vi "onStart.vi"(8 "error in (no error)":errorcluster, 11 "Camera":refnum<class "Camera.lvclass">) -> (0 "error out":errorcluster, 3 "Camera out":refnum<class "Camera.lvclass">)   [LabVIEW 2013, in "Camera.lvclass"]
doc: "JKI State Machine Objects (SMO) 1.0.4.18\nJKI - JKI\nCopyright (c) 2016, JKI"
uses:
  Camera.lvclass
  <vilib>/JKI/JKI SMO/SMO/SMO.lvclass
panel:
  # "For instructions on how to use the JKI State Machine Objects, examples and video tutorials, visit:\nhttp://jki.net/state-machine-objects/\n\nJKI State Machine Objects™\nhttp://jki.net/state-machine-objects/\nCopyright (C) 2005-2015, JKI <info@jki.net>\nALL RIGHTS RESERVED"
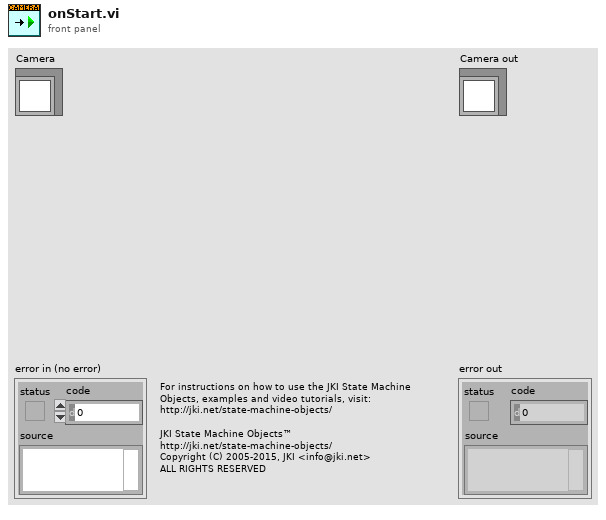
[diagram p1: front panel]
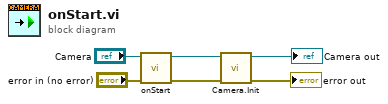
[diagram p0: block diagram]
diagram:
  n1 = call-parent "onStart.vi"("error in (no error)"="error in (no error)", "SMO"="Camera") -> ("error out"=w2:errorcluster, "SMO out"=w4:refnum<class "Camera.lvclass">)  [unwired: 8 in]
  n2 = call-dynamic "Camera.Init.vi"("error in (no error)"=w2, "Camera"=w4) -> ("error out"=→"error out":errorcluster, "Camera out"=→"Camera out":refnum<class "Camera.lvclass">)  [unwired: 8 in]
